vi "1B Dialog with Font Size control.vi"(8 "error in (no error)":errorcluster, 10 "T Button Name (\"OK\")":string="OK", 11 "message":string="message") -> (0 "error out":errorcluster, 3 "OK":bool)   [LabVIEW 2018]
panel:
  out "message":string
  in  "OK":bool
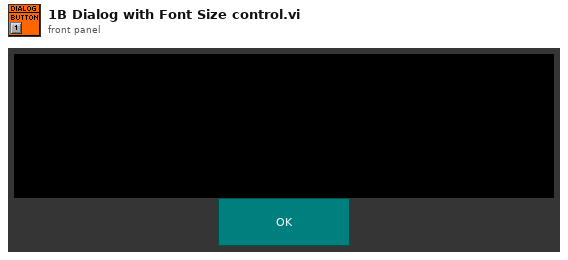
[diagram p1: front panel]
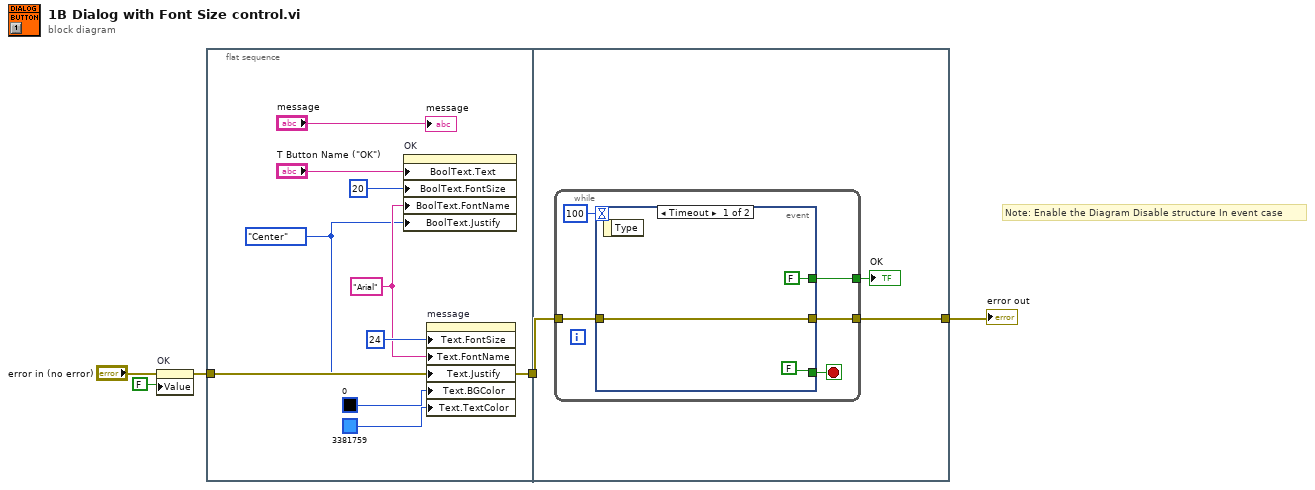
[diagram p0: block diagram]
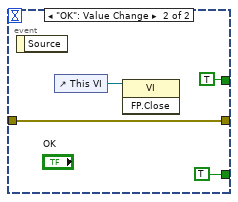
[diagram p2: hidden frame]
diagram:
  # "Note: Enable the Diagram Disable structure In event case"
  n1 = property on="OK" class="Bool (strict)"(error in="error in (no error)", "Value"=FALSE ("OK")) -> (error out=w2:errorcluster)  [unwired: 1 in, 1 out]
  n2 = flat-sequence {
    tunnel: [w12] -> w5
    tunnel: w2 -> [w12]
    tunnel: w5 -> [w16]
    tunnel: [w15] -> w4
    frame #0 {
      w8 = enum16{"Left", "Center", "Right"}."Center" ("Boolean Text.Justification")
      w9 = "Arial" ("Font Name")
      n3 = property on="OK" class="Bool"("BoolText.Text"="T Button Name (\"OK\")", "BoolText.FontSize"=u32 20 ("Boolean Text.Font:Size"), "BoolText.FontName"=w9, "BoolText.Justify"=w8) -> ()  [unwired: 2 in, 2 out]
      n4 = property on="message" class="Str"("Text.FontSize"=u32 24 ("Text.Font:Size"), "Text.FontName"=w9, "Text.Justify"=w8, "Text.BGColor"=u32 0, "Text.TextColor"=u32 3381759) -> ()  [unwired: 2 in, 2 out]
      "message" <- "message"
    }
    frame #1 {
      n5 = while {
        tunnel: [w20] -> w17
        tunnel: w16 -> [w18]
        tunnel: [w19] -> w15
        stop <- w21 stop-if-true
        n6 = event shown="[0] Timeout" {
          selector: _ -> [_ _]
          dyn-events: _ -> [_ _]
          timeout: 100 -> [_ _]
          tunnel: [FALSE TRUE] -> w21
          tunnel: [FALSE TRUE] -> w20
          tunnel: [w23 w27] -> w19
          tunnel: w18 -> [w23 w27]
          event Timeout {
            n7 = event-data() -> ()  [unwired: 2 out]
          }
          event "OK": Value Change {
            n8 = event-data() -> ()  [unwired: 2 out]
            n9 = control-ref of="This VI"() -> (w26:refnum<vi>)
            n10 = invoke class="VI" method="FP.Close"(reference=w26) -> ()  [unwired: 2 in, 3 out]
          }
        }
      }
      "OK" <- w17
    }
  }
  "error out" <- w4
